vi "Read Status.vi"(8 "error in (no error)":errorcluster, 11 "Transfer Group Status in":refnum<class "Transfer Group Status.lvclass">) -> (0 "error out":errorcluster, 2 "status":T1, 3 "Transfer Group Status out":refnum<class "Transfer Group Status.lvclass">)   [LabVIEW 2017, in "DSF Core.lvlib" / "Transfer Group Status.lvclass"]
uses:
  Transfer Group Status.lvclass
  C:/Program Files (x86)/National Instruments/LabVIEW 2017/vi.lib/NI/Memory Manager/Classes/Pointer/Pointer.lvclass
  Typedefs/DSF Transfer Group Status.ctl
  <vilib>/NI/Memory Manager/Classes/Pointer/Pointer.lvclass/Pointer.ctl
  <vilib>/NI/Memory Manager/Classes/Pointer/Errors.vi
  <vilib>/NI/Memory Manager/Classes/Pointer/Out of Bounds.vi
  <vilib>/NI/Memory Manager/Classes/Pointer/Get Size.vi
  <vilib>/NI/Memory Manager/VIs/Source.Write.String.vi
  <vilib>/NI/Memory Manager/Classes/Pointer/Write Pointer Size.vi
  <vilib>/NI/Memory Manager/Classes/Pointer/Create Error.vi
  <vilib>/NI/Memory Manager/VIs/Source.Write.Scalar.Base10.vi
  <vilib>/NI/Memory Manager/VIs/Source.Write.Scalar.Base10 (U64).vi
  <vilib>/NI/Memory Manager/VIs/New Error Cluster Constant.vi
  <vilib>/NI/Memory Manager/VIs/New Error Cluster Constant (512B).vi
  <vilib>/NI/Memory Manager/VIs/Error Cluster.Set Status.vi
  <vilib>/NI/Memory Manager/VIs/Error Cluster.Set Code.vi
  <vilib>/NI/Memory Manager/VIs/Error Cluster.Set VI Source.vi
  <vilib>/NI/Memory Manager/Constants/Constants.vi
  <vilib>/NI/Memory Manager/Constants/Library Name.vi
  <vilib>/NI/Memory Manager/Classes/Pointer/Pointer Error Info.vi
  <vilib>/NI/Memory Manager/Constants/Pointer Class Name.vi
  DSF Core.lvlib
  <vilib>/NI/Memory Manager/Classes/Pointer/Pointer.lvclass
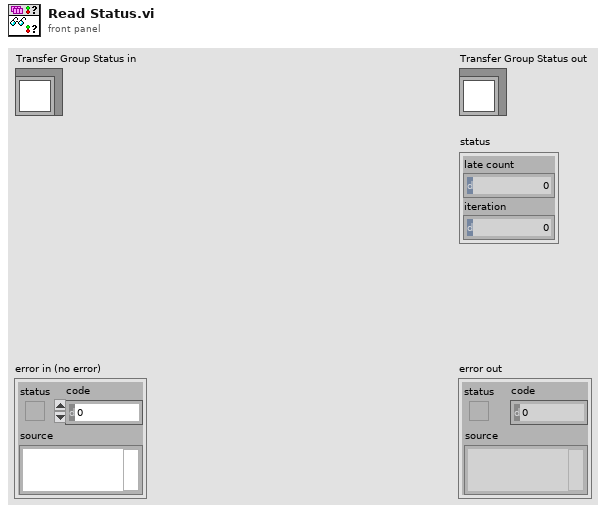
[diagram p1: front panel]
types:
  T1 = typedef "DSF Core.lvlib/DSF Transfer Group Status.ctl" = cluster{"late count":u64, "iteration":u64}
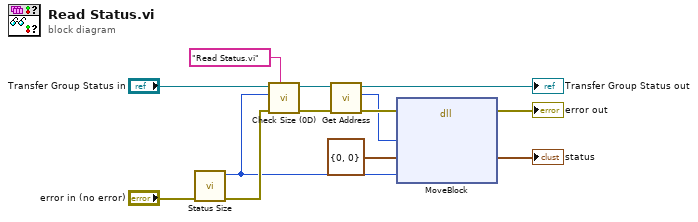
[diagram p0: block diagram]
diagram:
  n1 = call "Status Size.vi"("error in (no error)"="error in (no error)") -> ("error out"=w10:errorcluster, "size"=w7:u64)  [unwired: 9 in]
  n2 = call <vilib>:"Check Size (0D).vi"("source vi name"="Read Status.vi", "error in (no error)"=w10, "required size"=w7, "Pointer in"="Transfer Group Status in") -> ("error out"=w9:errorcluster, "Pointer out"=w12:refnum<class "Transfer Group Status.lvclass">)  [unwired: 5 in, 1 out]
  n3 = call <vilib>:"Get Address.vi"("Pointer in"=w12) -> ("address"=w8:u64, "Pointer out"=→"Transfer Group Status out":refnum<class "Transfer Group Status.lvclass">)  [unwired: 9 in]
  n4 = dll-call lib="LabVIEW" fn="MoveBlock"(error in=w9, "src"=w8, "dst"=T1 {"late count"=0, "iteration"=0} ("Transfer Group status"), "size"=w7) -> (error out=→"error out":errorcluster, "dst"=→"status":T1)  [unwired: 5 in, 1 out]
